vi "Write 32B RT FIFO.vi"(6 "overwrite on timeout (T)":bool, 7 "FIFO Debug Flags":refnum<class "Debug Flags FIFO.lvclass">, 8 "error in (no error)":errorcluster, 9 "timeout in ms (0)":i32, 10 "element":T2, 11 "RT FIFO in":T1) -> (0 "error out":errorcluster, 1 "timed out?":bool, 3 "RT FIFO out":T1)   [LabVIEW 2017, in "Data Sharing Framework Core.lvlib" / "Data Sharing Framework Engine.lvlib" / "Engine Interface.lvclass"]
uses:
  Engine Interface.lvclass
  32B Data.ctl
  32B Payload.ctl
  32B RT FIFO Reference.ctl
  Debug/Debug Flags FIFO/Debug Flags FIFO.lvclass
  Debug/Debug Flags FIFO/Debug Flags FIFO.lvclass/Debug Flags FIFO.ctl
panel:
  out "# elements":u32
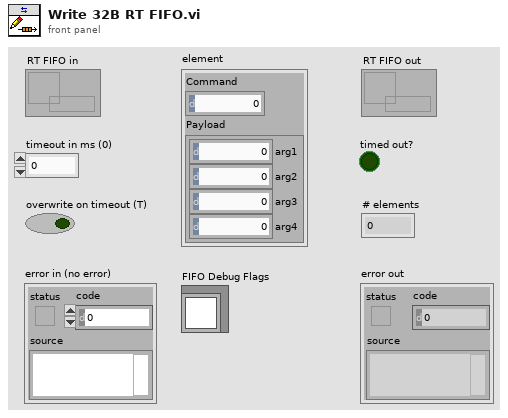
[diagram p1: front panel]
types:
  T1 = typedef "Data Sharing Framework Core.lvlib/Data Sharing Framework Engine.lvlib/Engine Interface.lvclass/32B RT FIFO Reference.ctl" = refnum<k33>
  T2 = typedef "Data Sharing Framework Core.lvlib/Data Sharing Framework Engine.lvlib/Engine Interface.lvclass/32B Data.ctl" = cluster{"Command":u8, "Payload":T3}
  T3 = typedef "Data Sharing Framework Core.lvlib/Data Sharing Framework Engine.lvlib/Engine Interface.lvclass/32B Payload.ctl" = cluster{"arg1":u64, "arg2":u64, "arg3":u64, "arg4":u64}
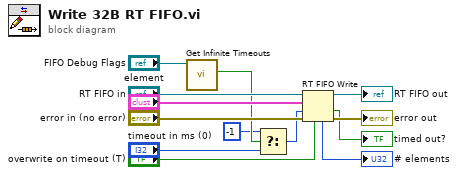
[diagram p0: block diagram]
diagram:
  n1 = call "Get Infinite Timeouts.vi"("FIFO Debug Flags in"="FIFO Debug Flags") -> ("infinite timeouts"=w2:bool)  [unwired: 9 in, 1 out]
  n2 = Select(t=-1, s=w2, f="timeout in ms (0)") -> (s? t:f=w3:i32)
  n3 = RT FIFO Write(0:"RT FIFO in", 1:"element", 2:w3, 3:"error in (no error)", 5:"overwrite on timeout (T)") -> (7:→"# elements":u32, 8:→"RT FIFO out":T1, 10:→"timed out?":bool, 11:→"error out":errorcluster)
